vi "SC10_enable_toggle.vi"(8 "error in (no error)":errorcluster, 11 "VISA resource name":refnum<visa-resource-name>) -> (0 "error out":errorcluster, 3 "VISA resource name out":refnum<visa-resource-name>)   [LabVIEW 2010]
panel:
  out "substring":string
  out "read buffer":string
  out "return count 3":u32
  out "return count":u32
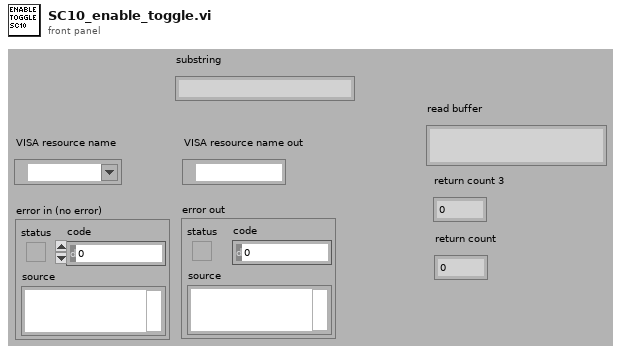
[diagram p1: front panel]
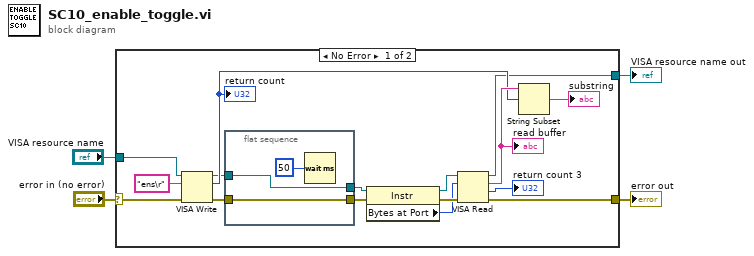
[diagram p0: block diagram]
diagram:
  n1 = case shown="No Error" "error in (no error)" {
    selector: "error in (no error)" -> [w20 w24]
    tunnel: [w6 w24] -> w3
    tunnel: [w5 w25] -> w2
    tunnel: "VISA resource name" -> [w19 w25]
    frame No Error {
      n2 = VISA Write(VISA resource name=w19, write buffer="ens\r", error in (no error)=w20) -> (VISA resource name out=w8:refnum<visa-resource-name>, return count=w9:u32, error out=w7:errorcluster)
      "return count" <- w9
      n3 = flat-sequence {
        tunnel: w8 -> [w22]
        tunnel: [w22] -> w12
        tunnel: w7 -> [w21]
        tunnel: [w21] -> w13
        frame #0 {
          n4 = Wait (ms)(milliseconds to wait=u32 50) -> ()  [unwired: 1 out]
        }
      }
      n5 = property class="Instr"(reference=w12, error in=w13) -> (reference out=w11:refnum<visa-resource-name>, error out=w14:errorcluster, "Bytes at Port"=w10:u32)
      n6 = VISA Read(VISA resource name=w11, byte count=w10, error in (no error)=w14) -> (VISA resource name out=w5:refnum<visa-resource-name>, read buffer=w16:string, return count=→"return count 3":u32, error out=w6:errorcluster)
      "read buffer" <- w16
      n7 = String Subset(string=w16, offset (0)=w9) -> (substring=→"substring":string)  [unwired: 1 in]
    }
    frame Error {
    }
  }
  "error out" <- w3
  "VISA resource name out" <- w2
